vi "createVirtualDrive.vi"(8 "error in (no error)":errorcluster, 11 "BuildWorker Controller in":refnum<class "BuildWorker Controller.lvclass">) -> (0 "error out":errorcluster, 3 "BuildWorker Controller out":refnum<class "BuildWorker Controller.lvclass">)   [LabVIEW 2017, in "BuildWorker Interface.lvlib" / "BuildWorker Controller.lvclass"]
uses:
  BuildWorker Controller.lvclass
  BuildWorker Controller.lvclass/BuildWorker Controller.ctl
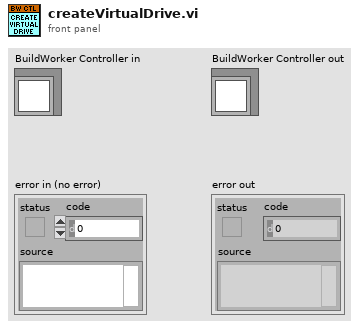
[diagram p1: front panel]
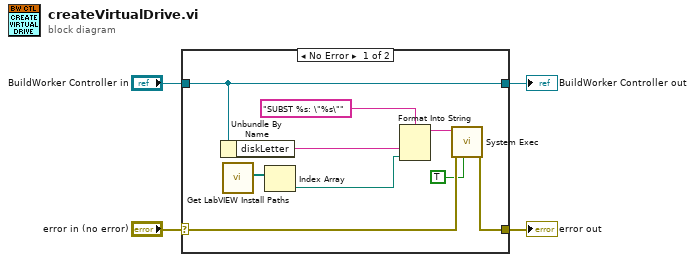
[diagram p0: block diagram]
diagram:
  n1 = case shown="No Error" "error in (no error)" {
    selector: "error in (no error)" -> [w9 w15]
    tunnel: [w8 w15] -> w3
    tunnel: [w13 w14] -> w1
    tunnel: "BuildWorker Controller in" -> [w13 w14]
    frame No Error {
      n2 = Unbundle By Name(w13) -> ("diskLetter"=w12:string)
      n3 = call "Get LabVIEW Install Paths.vi"() -> ("LV Directories"=w6:path[])  [unwired: 9 in, 2 out]
      n4 = Index Array(array=w6) -> (element=w5:path)  [unwired: 1 in]
      n5 = Format Into String(format string="SUBST %s: \"%s\"", w12, w5) -> (resulting string=w10:string)  [unwired: 2 in, 1 out]
      n6 = call <vilib>:"System Exec.vi"("run minimized? (F)"=TRUE, "error in (no error)"=w9, "command line"=w10) -> ("error out"=w8:errorcluster)  [unwired: 5 in, 3 out]
    }
    frame Error {
    }
  }
  "error out" <- w3
  "BuildWorker Controller out" <- w1
